vi "GetFullQualifierName.vi"(10 "file type":T1, 11 "File Path":path) -> (3 "FullQualifierName":string)   [LabVIEW 2020, in "DependencyChecker.lvlib"]
uses:
  DependencyChecker.lvlib
  <vilib>/Utility/lvfile.llb/FT_FileTypes.ctl
  <vilib>/Utility/lvfile.llb/NI_FileType.lvlib
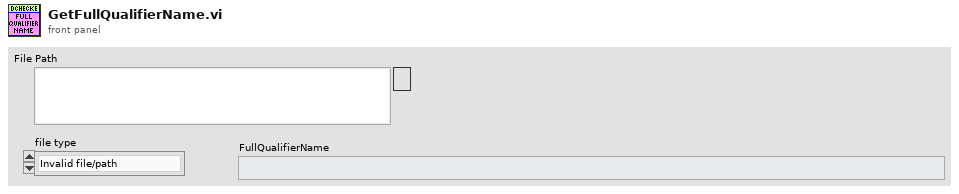
[diagram p1: front panel]
types:
  T1 = typedef "NI_FileType.lvlib/FT_FileTypes.ctl" = enum32{"Invalid file/path", "Unknown type", "Instrument", "Control", "Polymorphic VI", "Project", "Library", "LVClass", "XControl", "XNode", "CIN", "Run-time menu", "Palette menu", "LLB", "Shortcut", "Directory", "Class Private Data Control", "Statechart", "MathScript .m file", "Ladder Diagram", "LVLibp"}
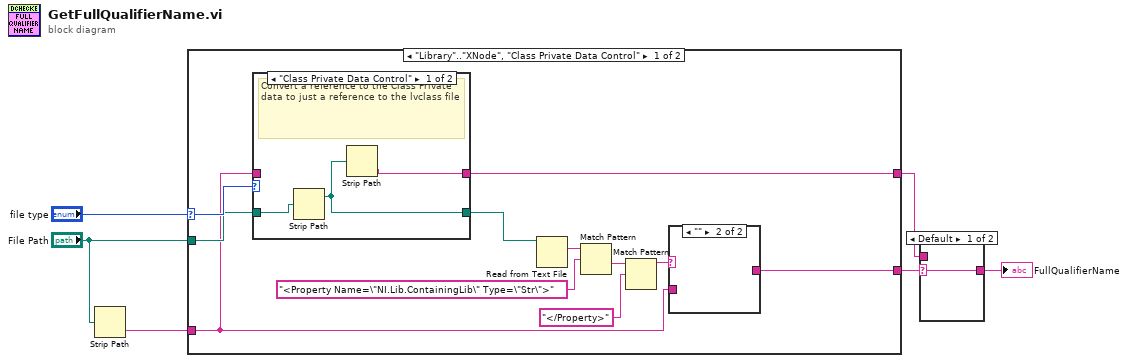
[diagram p0: block diagram]
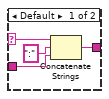
[diagram p2: hidden frame]
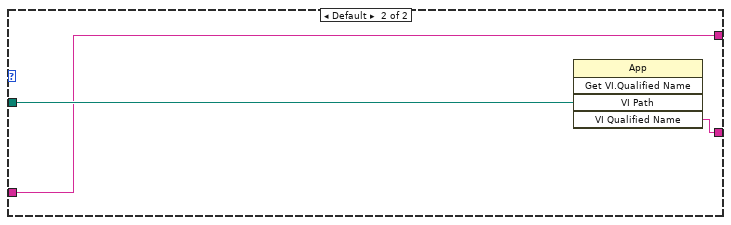
[diagram p4: hidden frame]
diagram:
  n1 = Strip Path(path="File Path") -> (name=w2:string)  [unwired: 1 out]
  n2 = case shown="\"Library\"..\"XNode\", \"Class Private Data Control\"" "file type" {
    selector: "file type" -> [w14 _]
    tunnel: "File Path" -> [w13 w29]
    tunnel: [w9 w28] -> w5
    tunnel: w2 -> [w8 w27]
    tunnel: [w7 w27] -> w1
    frame "Library".."XNode", "Class Private Data Control" {
      n3 = case shown="\"Class Private Data Control\"" w14 {
        tunnel: w13 -> [w24 w26]
        tunnel: [w23 w26] -> w12
        tunnel: w8 -> [_ w25]
        tunnel: [w22 w25] -> w7
        frame "Class Private Data Control" {
          # "Convert a reference to the Class Private data to just a reference to the lvclass file"
          n4 = Strip Path(path=w24) -> (stripped path=w23:path)  [unwired: 1 out]
          n5 = Strip Path(path=w23) -> (name=w22:string)  [unwired: 1 out]
        }
        frame Default {
        }
      }
      n6 = Read from Text File(file (use dialog)=w12) -> (text=w17:string)  [unwired: 3 in, 3 out]
      n7 = Match Pattern(string=w17, regular expression="<Property Name=\"NI.Lib.ContainingLib\" Type=\"Str\">") -> (after substring=w16:string)  [unwired: 1 in, 3 out]
      n8 = Match Pattern(string=w16, regular expression="</Property>") -> (before substring=w10:string)  [unwired: 1 in, 3 out]
      n9 = case shown="\"\"" w10 {
        selector: w10 -> [w19 _]
        tunnel: [w20 _] -> w9
        tunnel: w8 -> [w18 _]
        frame Default {
          n10 = Concatenate Strings(w19, ":" ("string"), w18) -> (w20:string)
        }
        frame "" {
        }
      }
    }
    frame Default {
      n11 = invoke class="App" method="Get VI.Qualified Name"("VI Path"=w29) -> ("VI Qualified Name"=w28:string)  [unwired: 4 in, 4 out]
    }
  }
  n12 = case shown="Default" w5 {
    selector: w5 -> [w30 _]
    tunnel: [w30 w31] -> w3
    tunnel: w1 -> [_ w31]
    frame Default {
    }
    frame "" {
    }
  }
  "FullQualifierName" <- w3
